vi "Lock IN and DC2200 Fluence Program.vi"() -> ()   [LabVIEW 2023]
uses:
  <vilib>/Analysis/1siggen.llb/Ramp Pattern by Samples.vi
  <vilib>/Analysis/baseanly.llb/Mean (DBL).vi
  <instrlib>/Stanford Research 830/Public/Data/Read (Multiple Points).vi
  <vilib>/Utility/file.llb/Write Delimited Spreadsheet (DBL).vi
  <instrlib>/Stanford Research 830/Stanford Research 830.lvlib
  <vilib>/Analysis/NI_AALBase.lvlib
panel:
  in  "type":u16(ring) items=["Linear", "Logarithmic"]
  in  "samples":i32=10
  in  "end":dbl=100.0 format="%0.2f"
  in  "start":dbl format="%0.2f"
  in  "Frequency (Hz)":dbl=90.0 caption="Frequency (20)"
  out "Current LED %":dbl=15806.315789473685
  in  "Current Min (0.0)":dbl
  in  "Laser Driver":refnum<visa-resource-name>="USB0::0x1313::0x80C8::M00982628::INSTR" caption="resource name"
  out "PV  vs. LED %":cluster{"Y":dbl[], "Y":dbl[]}[](graph)=[{"Y"=[20.0, 5282.105263157895, 10544.21052631579], "Y"=[0.1229557991027832, 0.0021543651819229126, 0.0013065412640571594]}]
  in  "Input Connection (0: Single-Ended Voltage)":u16(ring)=1 items=["Single-Ended Voltage", "Differential Voltage", "1 MOhm Current Gain", "100 MOhm Current Gain"]
  in  "file path (dialog if empty)":path=path "G:/.shortcut-targets-by-id/1Kj_JwS6Cfwfqaz0ugzl18DK49iv9Rs0M/Equipment + Data/Photocurrent Data + Drivers/Photoresponse Calibration/Si Thorlab PD in cryostat/Si Thorlab PD no gain unbiased LDR lockin.txt"
  in  "Lock in Average Number of Points (s)":u32=5
  in  "Lock-in Amp":refnum<visa-resource-name>="GPIB0::8::INSTR"
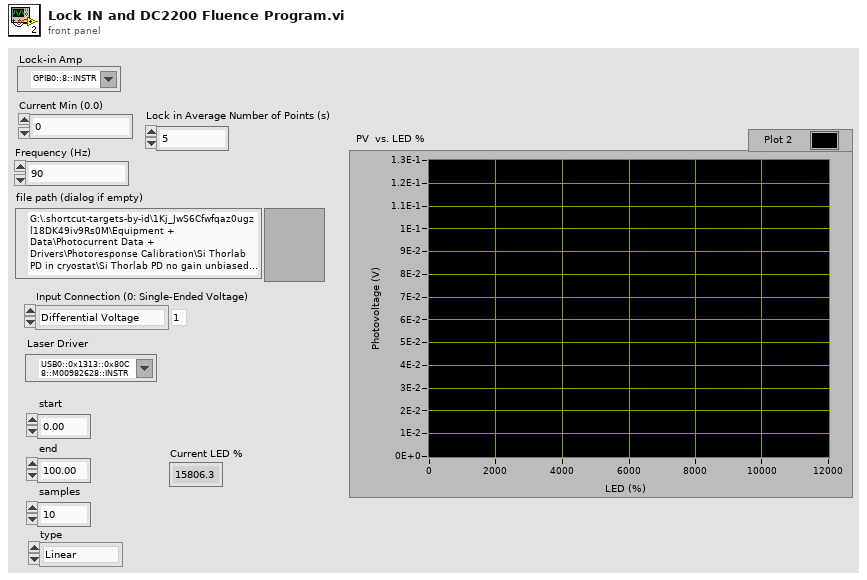
[diagram p1: front panel]
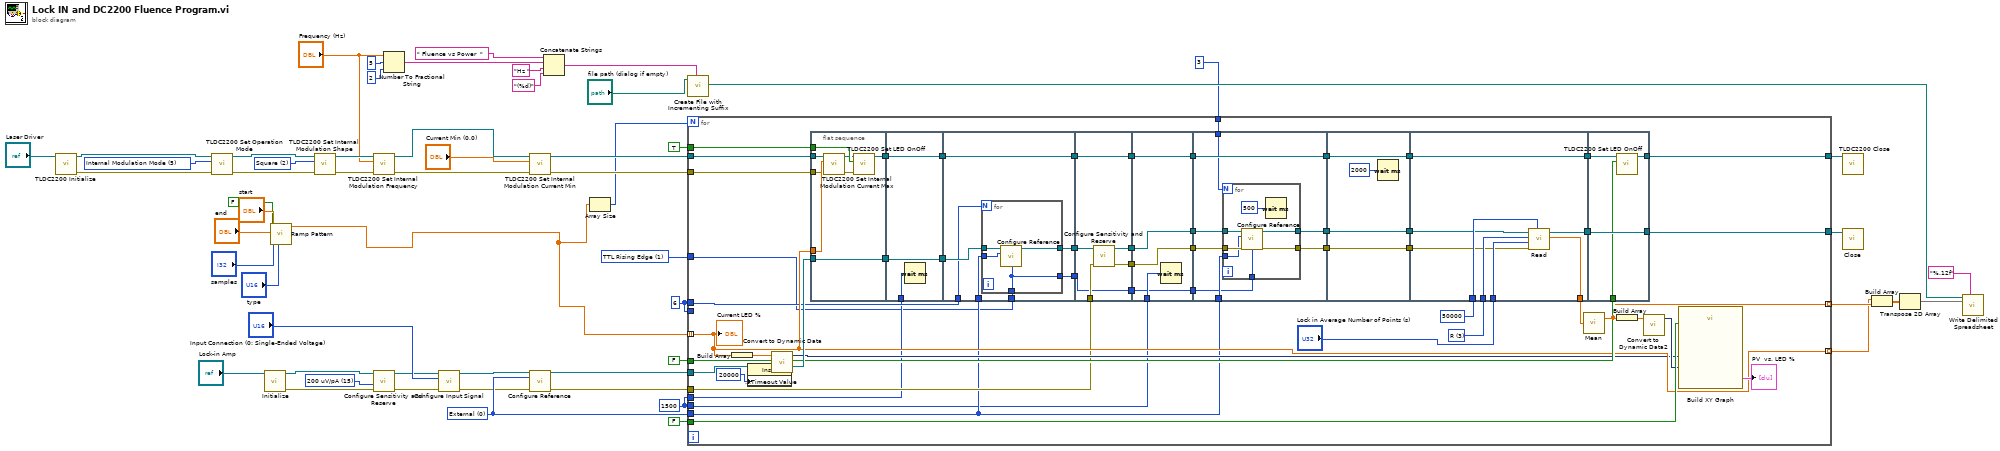
[diagram p0: block diagram]
diagram:
  w9 = u16 1 items=["Sine Zero Crossing", "TTL Rising Edge", "TTL Falling Edge"] ("External Reference Trigger (0: Sine Zero Crossing)")
  w22 = u32 1500 ("milliseconds to wait")
  w23 = 6
  w28 = u16 0 items=["External", "Internal"] ("Reference Source (1: Internal)")
  w40 = 5 items=["Constant Current Mode", "PWM Mode", "External Modulation Mode", "Brightness Mode", "Pulse Mode", "Internal Modulation Mode", "TTL Mode"] ("Operation Mode (Constant Current Mode)")
  w41 = 2 items=["Sine"=1, "Square"=2, "Triangle"=3] ("Shape (Sine)")
  w49 = i16 15 items=["Auto Gain"=-1, "2 nV/fA"=0, "5 nV/fA"=1, "10 nV/fA"=2, "20 nV/fA"=3, "50 nV/fA"=4, "100 nV/fA"=5, "200 nV/fA"=6, "500 nV/fA"=7, "1 uV/pA"=8, "2 uV/pA"=9, "5 uV/pA"=10, "10 uV/pA"=11, "20 uV/pA"=12, "50 uV/pA"=13, "100 uV/pA"=14, "200 uV/pA"=15, "500 uV/pA"=16, "1 mV/nA"=17, "2 mV/nA"=18, "5 mV/nA"=19, "10 mV/nA"=20, "20 mV/nA"=21, "50 mV/nA"=22, "100 mV/nA"=23, "200 mV/nA"=24, "500 mV/mA"=25, "1 V/uA"=26] ("Sensitivity (-1: Auto gain)")
  n1 = call <instrlib>:"TLDC2200 Initialize.vi"("resource name"="Laser Driver") -> ("error out"=w47:errorcluster, "instrument handle out"=w46:refnum<visa-resource-name>)  [unwired: 9 in]
  n2 = call <instrlib>:"TLDC2200 Set Operation Mode.vi"("error in (no error)"=w47, "Operation Mode (Constant Current Mode)"=w40, "instrument handle"=w46) -> ("error out"=w45:errorcluster, "instrument handle out"=w44:refnum<visa-resource-name>)  [unwired: 7 in]
  n3 = call <instrlib>:"Initialize.vi"("VISA resource name"="Lock-in Amp") -> ("error out"=w27:errorcluster, "VISA resource name out"=w51:refnum<visa-resource-name>)  [unwired: 9 in]
  n4 = call-poly <vilib>:"Ramp Pattern.vi"("type"="type", "exclude end?"=FALSE, "start"="start", "end"="end", "samples"="samples") -> ("Ramp Pattern"=w6:dbl[])  [unwired: 5 in, 1 out]
  n5 = call <instrlib>:"TLDC2200 Set Internal Modulation Shape.vi"("error in (no error)"=w45, "Shape (Sine)"=w41, "instrument handle"=w44) -> ("error out"=w43:errorcluster, "instrument handle out"=w42:refnum<visa-resource-name>)  [unwired: 7 in]
  n6 = call <instrlib>:"TLDC2200 Set Internal Modulation Frequency.vi"("error in (no error)"=w43, "Frequency (20)"="Frequency (Hz)", "instrument handle"=w42) -> ("error out"=w20:errorcluster, "instrument handle out"=w21:refnum<visa-resource-name>)  [unwired: 7 in]
  n7 = call <instrlib>:"Configure Sensitivity and Reserve.vi"("error in (no error)"=w27, "Sensitivity (-1: Auto gain)"=w49, "VISA resource name"=w51) -> ("error out"=w26:errorcluster, "VISA resource name out"=w50:refnum<visa-resource-name>)  [unwired: 7 in]
  n8 = Number To Fractional String(number="Frequency (Hz)", width (-)=i16 5, precision (6)=i16 2) -> (F-format string=w13:string)  [unwired: 1 in]
  n9 = call <instrlib>:"Configure Input Signal.vi"("error in (no error)"=w26, "Input Connection (0: Single-Ended Voltage)"="Input Connection (0: Single-Ended Voltage)", "VISA resource name"=w50) -> ("error out"=w25:errorcluster, "VISA resource name out"=w31:refnum<visa-resource-name>)  [unwired: 7 in]
  n10 = call <instrlib>:"TLDC2200 Set Internal Modulation Current Min.vi"("error in (no error)"=w20, "Current Min (0.0)"="Current Min (0.0)", "instrument handle"=w21) -> ("error out"=w33:errorcluster, "instrument handle out"=w34:refnum<visa-resource-name>)  [unwired: 7 in]
  n11 = call <instrlib>:"Configure Reference.vi"("VISA resource name"=w31, "Reference Source (1: Internal)"=w28, "error in (no error)"=w25) -> ("VISA resource name out"=w30:refnum<visa-resource-name>, "error out"=w24:errorcluster)  [unwired: 11 in]
  n12 = Concatenate Strings(" Fluence vs Power  " ("string"), w13, "Hz " ("string"), "(%d)" ("string")) -> (w19:string)
  n13 = Array Size(array=w6) -> (size(s)=w7:i32)
  n14 = call <vilib>:"Create File with Incrementing Suffix.vi"("format string (\" (%d)\")"=w19, "file path"="file path (dialog if empty)") -> ("actual path"=w11:path)  [unwired: 7 in, 2 out]
  n15 = for {
    N: w7 -> [_]
    tunnel: [w101] -> w56
    tunnel: w6 -> [w89] mode=indexing
    tunnel: [w91] -> w48 mode=indexing
    tunnel: TRUE ("LED On/Off (Off)") -> [w107]
    tunnel: FALSE ("LED On/Off (Off)") -> [w99]
    tunnel: [w98] -> w37
    tunnel: w34 -> [w97]
    tunnel: [w89] -> w35 mode=indexing
    tunnel: w33 -> [w95]
    tunnel: w30 -> [w94]
    tunnel: FALSE ("Reset") -> [w93]
    tunnel: w28 -> [w69]
    tunnel: w24 -> [w85]
    tunnel: w23 -> [_]
    tunnel: w23 -> [w70]
    tunnel: w22 -> [w64]
    tunnel: w22 -> [w63]
    tunnel: w9 -> [w62]
    tunnel: 3 -> [w58]
    w103 = u16 3 items=["X"=1, "Y"=2, "R"=3, "Theta"=4, "Channel 1"=5, "Channel 2"=6, "Aux In 1"=7, "Aux In 2"=8, "Aux In 3"=9, "Aux In 4"=10] ("Parameter (1: X)")
    n16 = Build Array(w89) -> (w88:dbl[])
    n17 = property class="Instr"(reference=w94, "General Settings:Timeout Value"=u32 20000) -> (reference out=w106:refnum<visa-resource-name>)  [unwired: 1 in, 1 out]
    n18 = call "Convert to Dynamic Data"("Array"=w88) -> ("Dynamic Data Type"=w86:dynamicdata)  [unwired: 3 in]
    n19 = flat-sequence {
      tunnel: w89 -> [w112]
      tunnel: w107 -> [w116]
      tunnel: [w115] -> w68
      tunnel: w106 -> [w115]
      tunnel: w97 -> [w113]
      tunnel: [w114] -> w66
      tunnel: w95 -> [w111]
      tunnel: w68 -> [w119]
      tunnel: [w119] -> w67
      tunnel: w66 -> [w118]
      tunnel: [w118] -> w65
      tunnel: w64 -> [w117]
      tunnel: w67 -> [w125]
      tunnel: [w124] -> w72
      tunnel: w65 -> [w126]
      tunnel: [w126] -> w71
      tunnel: w70 -> [w123]
      tunnel: w69 -> [w122]
      tunnel: w62 -> [w121]
      tunnel: [w120] -> w59
      tunnel: w72 -> [w132]
      tunnel: [w136] -> w84
      tunnel: w71 -> [w136]
      tunnel: [w135] -> w82
      tunnel: [w134] -> w80
      tunnel: w85 -> [w133]
      tunnel: [w131] -> w60
      tunnel: w59 -> [w131]
      tunnel: w84 -> [w141]
      tunnel: [w141] -> w83
      tunnel: w82 -> [w140]
      tunnel: [w140] -> w81
      tunnel: w80 -> [w139]
      tunnel: [w139] -> w79
      tunnel: w63 -> [w138]
      tunnel: [w137] -> w61
      tunnel: w60 -> [w137]
      tunnel: [w147] -> w78
      tunnel: [w149] -> w76
      tunnel: w83 -> [w149]
      tunnel: w81 -> [w148]
      tunnel: w69 -> [w144]
      tunnel: w79 -> [w146]
      tunnel: [w145] -> w74
      tunnel: w61 -> [w143]
      tunnel: w58 -> [w142]
      tunnel: w78 -> [w160]
      tunnel: [w160] -> w77
      tunnel: w76 -> [w159]
      tunnel: [w159] -> w75
      tunnel: w74 -> [w158]
      tunnel: [w158] -> w73
      tunnel: u32 50000 ("Maximum Time (10000 ms)") -> [w168]
      tunnel: "Lock in Average Number of Points (s)" -> [w167]
      tunnel: w103 -> [w166]
      tunnel: [w165] -> w102
      tunnel: w77 -> [w163]
      tunnel: [w164] -> w100
      tunnel: [w162] -> w96
      tunnel: w75 -> [w162]
      tunnel: w73 -> [w161]
      tunnel: [w172] -> w101
      tunnel: w100 -> [w172]
      tunnel: w99 -> [w171]
      tunnel: [w170] -> w98
      tunnel: w96 -> [w169]
      frame #0 {
        n20 = call <instrlib>:"TLDC2200 Set Internal Modulation Current Max.vi"("error in (no error)"=w111, "Current Max (0.0)"=w112, "instrument handle"=w113) -> ("error out"=w109:errorcluster, "instrument handle out"=w110:refnum<visa-resource-name>)  [unwired: 7 in]
        n21 = call <instrlib>:"TLDC2200 Set LED OnOff.vi"("error in (no error)"=w109, "LED On/Off (Off)"=w116, "instrument handle"=w110) -> ("instrument handle out"=w114:refnum<visa-resource-name>)  [unwired: 7 in, 1 out]
      }
      frame #1 {
        n22 = Wait (ms)(milliseconds to wait=w117) -> ()  [unwired: 1 out]
      }
      frame #2 {
        n23 = for {
          N: w123 -> [_]
          tunnel: w125 -> [w130]
          tunnel: [w129] -> w124
          tunnel: w122 -> [w128]
          tunnel: w121 -> [w127]
          tunnel: [w127] -> w120
          n24 = call <instrlib>:"Configure Reference.vi"("VISA resource name"=w130, "Reference Source (1: Internal)"=w128, "External Reference Trigger (0: Sine Zero Crossing)"=w127) -> ("VISA resource name out"=w129:refnum<visa-resource-name>)  [unwired: 11 in, 1 out]
        }
      }
      frame #3 {
        n25 = call <instrlib>:"Configure Sensitivity and Reserve.vi"("error in (no error)"=w133, "VISA resource name"=w132) -> ("error out"=w134:errorcluster, "VISA resource name out"=w135:refnum<visa-resource-name>)  [unwired: 8 in]
      }
      frame #4 {
        n26 = Wait (ms)(milliseconds to wait=w138) -> ()  [unwired: 1 out]
      }
      frame #5 {
        n27 = for {
          N: w142 -> [_]
          tunnel: w148 -> [w156]
          tunnel: [w155] -> w147
          tunnel: w146 -> [w154]
          tunnel: [w153] -> w145
          tunnel: w144 -> [w151]
          tunnel: w143 -> [w150]
          n28 = call <instrlib>:"Configure Reference.vi"("VISA resource name"=w156, "Reference Source (1: Internal)"=w151, "error in (no error)"=w154, "External Reference Trigger (0: Sine Zero Crossing)"=w150) -> ("VISA resource name out"=w155:refnum<visa-resource-name>, "error out"=w153:errorcluster)  [unwired: 10 in]
          n29 = Wait (ms)(milliseconds to wait=u32 500) -> ()  [unwired: 1 out]
        }
      }
      frame #6 {
        n30 = Wait (ms)(milliseconds to wait=u32 2000) -> ()  [unwired: 1 out]
      }
      frame #7 {
        n31 = call-poly <instrlib>:"Read.vi"("Maximum Time (10000 ms)"=w168, "error in (no error)"=w161, "Number of Points (100)"=w167, "Channel (1: Channel 1 Display)"=w166, "VISA resource name"=w163) -> ("Measurements"=w165:sgl[], "VISA resource name out"=w164:refnum<visa-resource-name>)  [unwired: 4 in, 1 out]
      }
      frame #8 {
        n32 = call <instrlib>:"TLDC2200 Set LED OnOff.vi"("LED On/Off (Off)"=w171, "instrument handle"=w169) -> ("instrument handle out"=w170:refnum<visa-resource-name>)  [unwired: 8 in, 1 out]
      }
    }
    n33 = call-poly <vilib>:"Mean.vi"("X"=w102) -> ("mean"=w91:dbl)  [unwired: 1 out]
    n34 = Build Array(w91) -> (w90:dbl[])
    n35 = call "Convert to Dynamic Data2"("Array"=w90) -> ("Dynamic Data Type"=w87:dynamicdata)  [unwired: 3 in]
    n36 = call "Build XY Graph"("Reset"=w93, "Y Input"=w87, "X Input"=w86) -> ("XY Graph"=→"PV  vs. LED %":cluster{"Y":dbl[], "Y":dbl[]}[])  [unwired: 7 in, 1 out]
    "Current LED %" <- w89
  }
  n37 = call <instrlib>:"TLDC2200 Close.vi"("instrument handle"=w37) -> ()  [unwired: 10 in, 1 out]
  n38 = call <instrlib>:"Close.vi"("VISA resource name"=w56) -> ()  [unwired: 10 in, 1 out]
  n39 = Build Array(w35, w48) -> (w54:dbl[][])
  n40 = Transpose 2D Array(2D array=w54) -> (transposed array=w53:dbl[][])
  n41 = call-poly <vilib>:"Write Delimited Spreadsheet.vi"("file path (dialog if empty)"=w11, "format (%.3f)"="%.12f", "2D data"=w53) -> ()  [unwired: 11 in, 2 out]
